vi "Unpack Pixels (SubVI).vi"(11 "Image Array (64 Bit)":u64[](array[numeric])) -> (3 "Image Array (8 Bit)":u8[](array[numeric]))   [LabVIEW 2015]
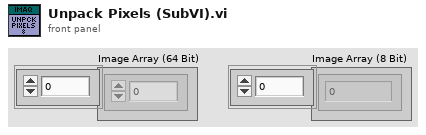
[diagram p1: front panel]
types:
  T1 = enum16{"big-endian, network order", "native, host order", "little-endian"}
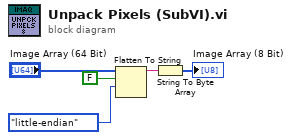
[diagram p0: block diagram]
diagram:
  n1 = Flatten To String(anything="Image Array (64 Bit)", prepend array or string size? (T)=FALSE, byte order (0:big-endian, network order)=T1."little-endian") -> (data string=w5:string)  [unwired: 1 in, 2 out]
  n2 = String To Byte Array(string=w5) -> (unsigned byte array=→"Image Array (8 Bit)":u8[])
